vi "Purge Queue.vi"(8 "error in (no error)":errorcluster, 11 "SQS in":refnum<class "NI_AWS_SQS.lvclass">) -> (0 "error out":errorcluster, 3 "SQS out":refnum<class "NI_AWS_SQS.lvclass">)   [LabVIEW 2015, in "NI_AWS_SQS.lvclass"]
uses:
  NI_AWS_SQS.lvclass
  Core/Name Value Pair.ctl
  Core/Request Options.ctl
  NI_AWS_SQS.lvclass/NI_AWS_SQS.ctl
  Read Account Number.vi
  Read Name.vi
  Core/NI_AWS_Core.lvclass
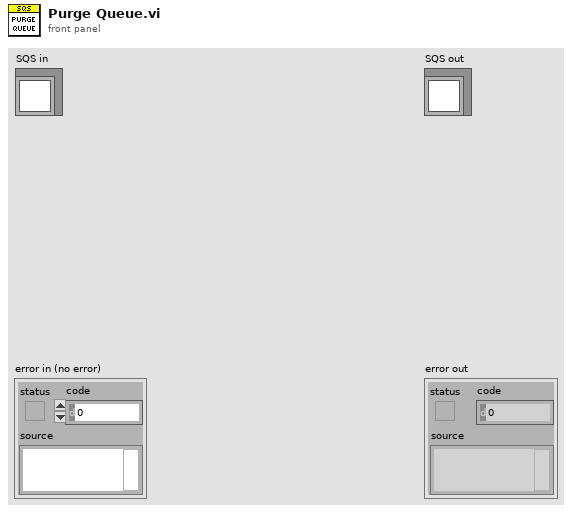
[diagram p1: front panel]
types:
  T1 = typedef "NI_AWS_Core.lvclass/Request Options.ctl" = cluster{"request headers":T2[], "request parameters":T2[], "request body":string}
  T2 = typedef "NI_AWS_Core.lvclass/Name Value Pair.ctl" = cluster{"name":string, "value":string}
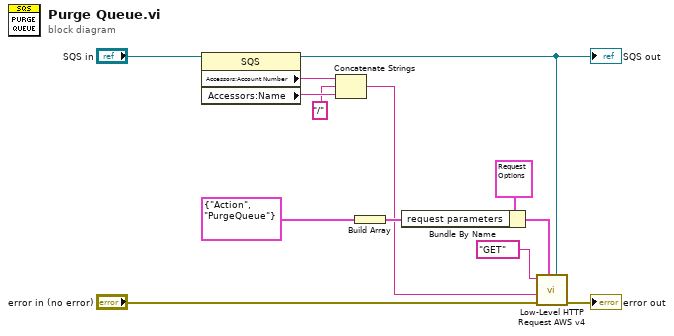
[diagram p0: block diagram]
diagram:
  n1 = property class="SQS"(reference="SQS in") -> (reference out=w6:refnum<class "NI_AWS_SQS.lvclass">, "Accessors:Account Number"=w5:string, "Accessors:Name"=w4:string)  [unwired: 1 in, 1 out]
  "SQS out" <- w6
  n2 = Concatenate Strings(w5, "/", w4) -> (w2:string)
  n3 = Build Array(T2 {"name"="Action", "value"="PurgeQueue"} ("Cluster")) -> (w7:T2[])
  n4 = Bundle By Name(cluster=T1 {"request headers"=[], "request parameters"=[{"name"="Action", "value"="ListQueues"}], "request body"=""} ("Request Options"), "request parameters"=w7) -> (w8:T1)
  n5 = call "Low-Level HTTP Request AWS v4.vi"("AWS Core"=w6, "Request Options"=w8, "error in (no error)"="error in (no error)", "URL Suffix"=w2, "HTTP-Verb"="GET") -> ("error out"=→"error out":errorcluster)  [unwired: 4 in, 2 out]
